vi "Write 1D Double.vi"(8 "error in":errorcluster, 9 "Write/Read Cell Numeric":T1 {"Data 1D" format="%.2f"; "Data 2D" format="%.2f"; "1 Data" format="%.2f"}, 11 "Work Sheet 2":refnum<k7>) -> (0 "error out":errorcluster, 3 "Work Sheet":refnum<k7>)   [LabVIEW 2017]
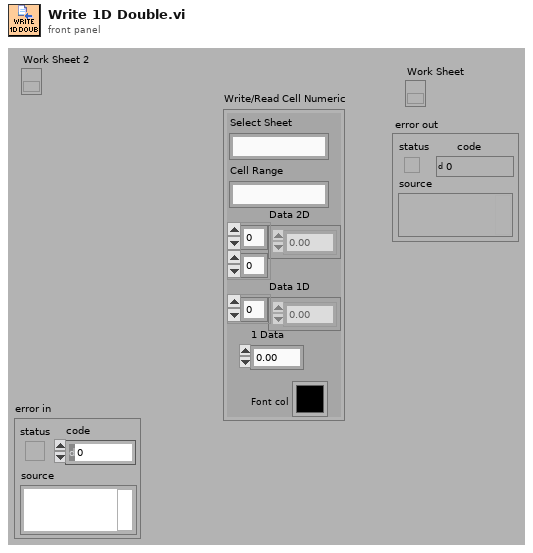
[diagram p1: front panel]
types:
  T1 = cluster{"Cell Range":string, "Select Sheet":string, "1 Data":dbl, "Data 2D":dbl[][], "Data 1D":dbl[], "Font col":u32}
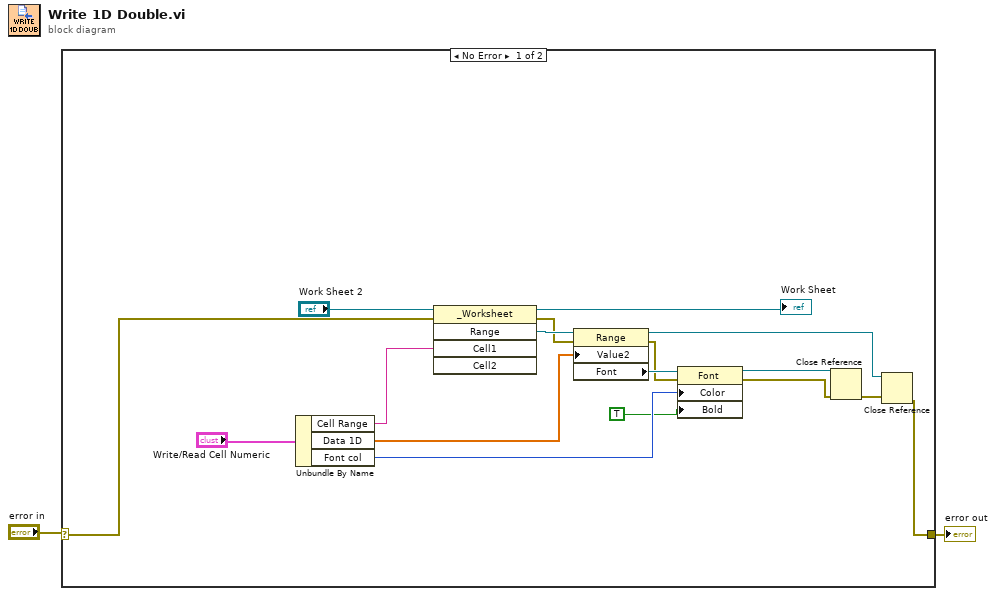
[diagram p0: block diagram]
diagram:
  n1 = case shown="No Error" "error in" {
    selector: "error in" -> [w18 w20]
    tunnel: [w4 w20] -> w1
    frame No Error {
      n2 = Unbundle By Name("Write/Read Cell Numeric") -> ("Cell Range"=w13:string, "Data 1D"=w14:dbl[], "Font col"=w10:u32)
      n3 = invoke class="_Worksheet" method="Range"(reference="Work Sheet 2", error in=w18, "Cell1"=w13) -> (reference out=→"Work Sheet":refnum<k7>, error out=w17:errorcluster, "Range"=w19:refnum<k7>)  [unwired: 2 in, 2 out]
      n4 = property class="Range"(reference=w19, error in=w17, "Value2"=w14) -> (reference out=w5:refnum<k7>, error out=w9:errorcluster, "Font"=w11:refnum<k7>)
      n5 = property class="Font"(reference=w11, error in=w9, "Color"=w10, "Bold"=TRUE) -> (reference out=w7:refnum<k7>, error out=w8:errorcluster)
      n6 = Close Reference(reference=w7, error in (no error)=w8) -> (error out=w6:errorcluster)
      n7 = Close Reference(reference=w5, error in (no error)=w6) -> (error out=w4:errorcluster)
    }
    frame Error {
    }
  }
  "error out" <- w1
